vi "call async imaq save.vi"(7 "Status":T1, 8 "error in (no error)":errorcluster, 9 "Boolean":bool, 10 "Refnum in":T2, 11 "FakeCamera in":refnum<class "Point Grey Camera.lvclass">) -> (0 "error out":errorcluster, 3 "FakeCamera out":refnum<class "Point Grey Camera.lvclass">)   [LabVIEW 2020, in "Point Grey Camera.lvclass"]
uses:
  Point Grey Camera.lvclass
  <vilib>/vision/Image Controls.llb/IMAQ Image.ctl
  subVis/1st or last shot of scan.ctl
panel:
  out "F-format string":string
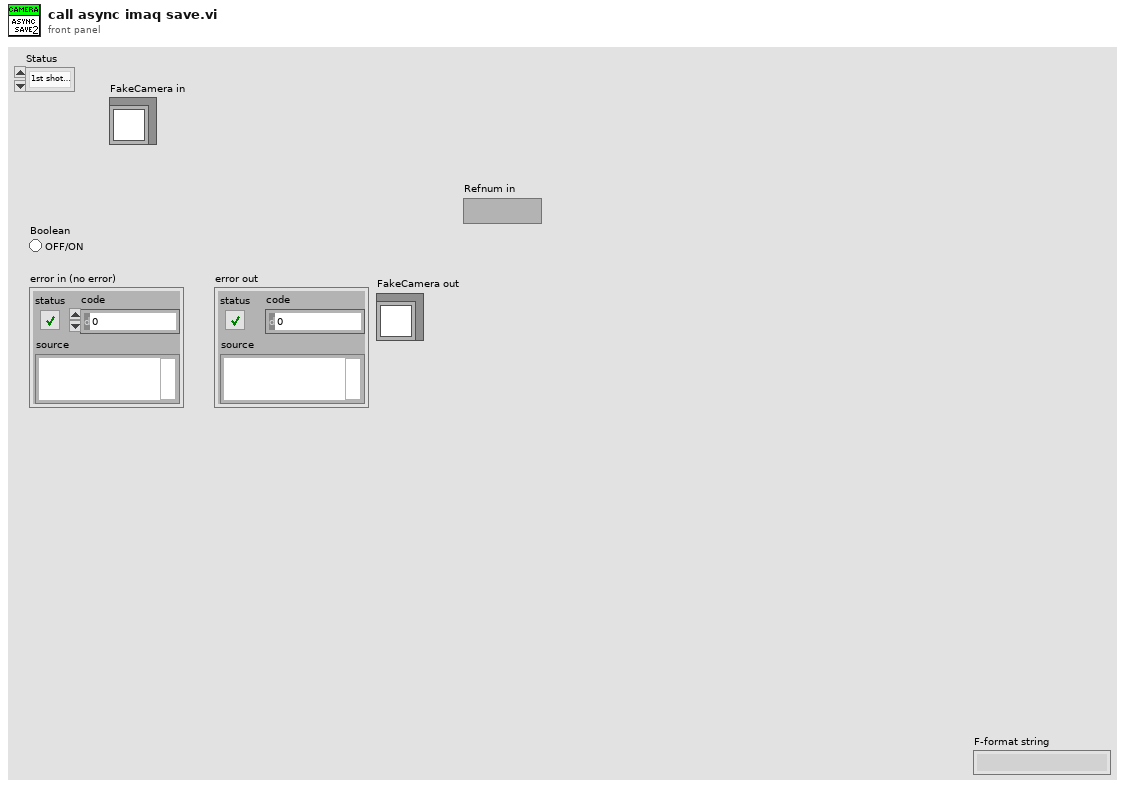
[diagram p1: front panel]
types:
  T1 = typedef "1st or last shot of scan.ctl" = enum16{"1st shot of scan", "1st shot after scan end", "other"}
  T2 = typedef "IMAQ Image.ctl" = refnum<image>
  T3 = typedef "Image Type" = u32
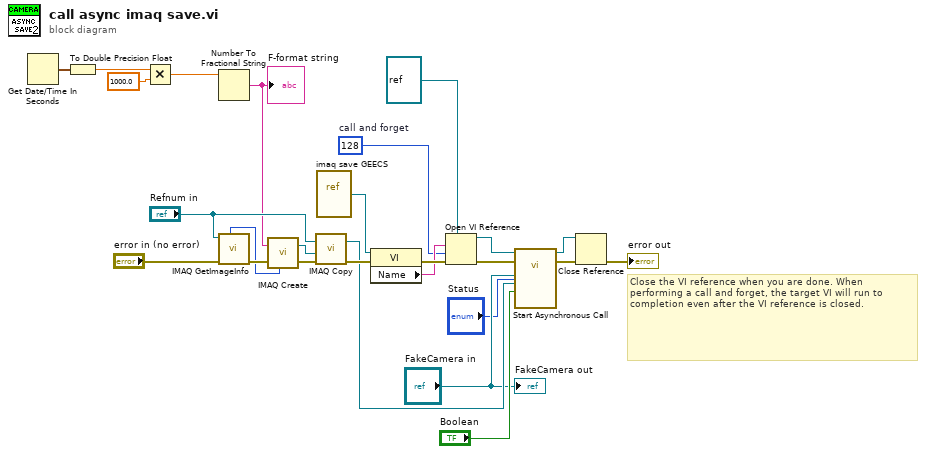
[diagram p0: block diagram]
diagram:
  w12 = 128  # call and forget
  # "Close the VI reference when you are done. When performing a call and forget, the target VI will run to completion even after the VI reference is closed."
  n1 = Get Date/Time In Seconds() -> (seconds since 1Jan1904=w5:timestamp)
  n2 = To Double Precision Float(number=w5) -> (double precision float=w4:dbl)
  n3 = Multiply(x=w4, y=1000.0) -> (x*y=w3:dbl)
  n4 = Number To Fractional String(number=w3) -> (F-format string=w1:string)  [unwired: 3 in]
  "F-format string" <- w1
  n5 = call "IMAQ GetImageInfo"("error in (no error)"="error in (no error)", "Image"="Refnum in") -> ("error out"=w24:errorcluster, "Image Type"=w9:T3)  [unwired: 2 in, 6 out]
  n6 = call "IMAQ Create"("Image Name"=w1, "Image Type"=w9, "error in (no error)"=w24) -> ("New Image"=w10:T2, "error out"=w25:errorcluster)  [unwired: 2 in]
  n7 = call "IMAQ Copy"("error in (no error)"=w25, "Image Dst"=w10, "Image Src"="Refnum in") -> ("error out"=w26:errorcluster, "Image Dst Out"=w8:T2)  [unwired: 3 in]
  n8 = vi-ref "imaq save GEECS.vi"() -> (w18:refnum<vi>)
  n9 = property class="VI"(reference=w18, error in=w26) -> (error out=w20:errorcluster, "Name"=w19:string)  [unwired: 1 out]
  n10 = Open VI Reference(type specifier VI Refnum (for type only)=refnum<vi> refnum, vi path=w19, options=w12, error in (no error)=w20) -> (vi reference=w14:refnum<vi>, error out=w15:errorcluster)  [unwired: 2 in]
  n11 = call-by-ref "Start Asynchronous Call"(reference=w14, error in=w15, "Status"="Status", "file already written"="Boolean", "Refnum in"=w8, "FakeCamera in"="FakeCamera in") -> (reference out=w17:refnum<vi>, error out=w16:errorcluster)  [unwired: 6 in, 2 out]
  n12 = Close Reference(reference=w17, error in (no error)=w16) -> (error out=→"error out":errorcluster)
  "FakeCamera out" <- "FakeCamera in"
